vi "excel_lectura_archivo.vi"(8 "error in (no error)":errorcluster, 10 "referencia excel in":refnum<file>) -> (0 "error out":errorcluster, 1 "array_grados":i64[][](array[numeric]), 2 "referencia excel out":refnum<file>, 3 "ruta excel out":path)   [LabVIEW 2026]
uses:
  <vilib>/Utility/file.llb/Read Delimited Spreadsheet (I64).vi
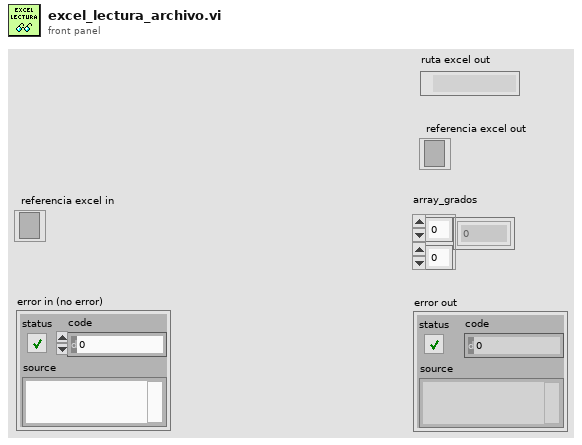
[diagram p1: front panel]
types:
  T1 = enum16{"open", "replace", "create", "open or create", "replace or create", "replace or create with confirmation"}
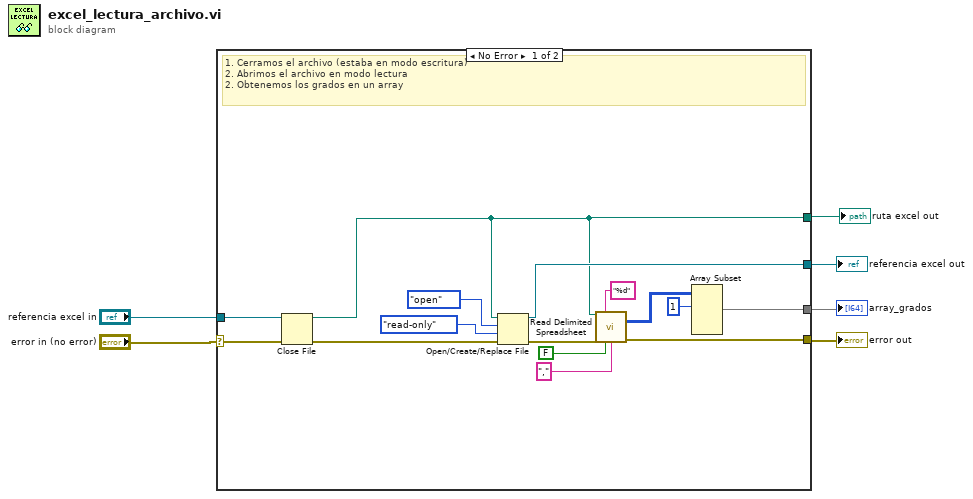
[diagram p0: block diagram]
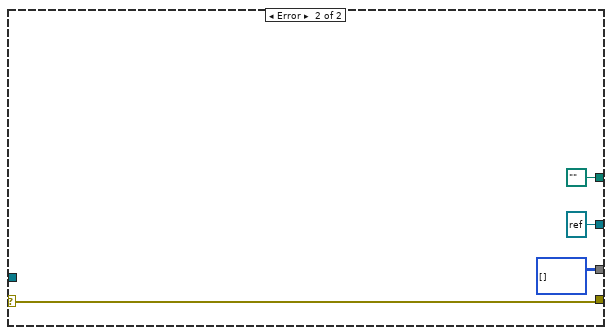
[diagram p2: hidden frame]
diagram:
  n1 = case shown="No Error" "error in (no error)" {
    selector: "error in (no error)" -> [w12 w25]
    tunnel: [w16 w25] -> w6
    tunnel: [w13 i64[][] []] -> w3
    tunnel: [w8 path "" ("ruta excel in")] -> w4
    tunnel: "referencia excel in" -> [w10 _]
    tunnel: [w9 refnum<file> refnum ("refnum out")] -> w1
    frame No Error {
      # "1. Cerramos el archivo (estaba en modo escritura)\n2. Abrimos el archivo en modo lectura\n2. Obtenemos los grados en un array"
      n2 = Close File(refnum=w10, error in=w12) -> (path=w8:path, error out=w11:errorcluster)
      n3 = Open/Create/Replace File(file path (use dialog)=w8, error in=w11, operation (0:open)=T1."open", access (0:read/write)=enum16{"read/write", "read-only", "write-only"}."read-only") -> (refnum out=w9:refnum<file>, error out=w19:errorcluster)  [unwired: 2 in, 1 out]
      n4 = call-poly <vilib>:"Read Delimited Spreadsheet.vi"("file path (dialog if empty)"=w8, "format (%d)"="%d", "error in (no error)"=w19, "transpose? (F)"=FALSE, "delimiter (\\t)"="," ("delimiter (\\t)")) -> ("all rows"=w15:i64[][], "error out"=w16:errorcluster)  [unwired: 5 in, 4 out]
      n5 = Array Subset(array=w15, index (row)=1 ("index")) -> (w13:i64[][])  [unwired: 3 in]
    }
    frame Error {
    }
  }
  "error out" <- w6
  "ruta excel out" <- w4
  "array_grados" <- w3
  "referencia excel out" <- w1
